vi "Set Current UUT.vi"(8 "error in (no error)":errorcluster, 10 "Current UUT":u32, 11 "LED Board Visual Test in":refnum<class "LED Board Test.lvclass">) -> (0 "error out":errorcluster, 3 "LED Board Visual Test out":refnum<class "LED Board Test.lvclass">)   [LabVIEW 2015, in "LED Board Test.lvclass"]
uses:
  LED Board Test.lvclass
  LED Board Test.lvclass/LED Board Test.ctl
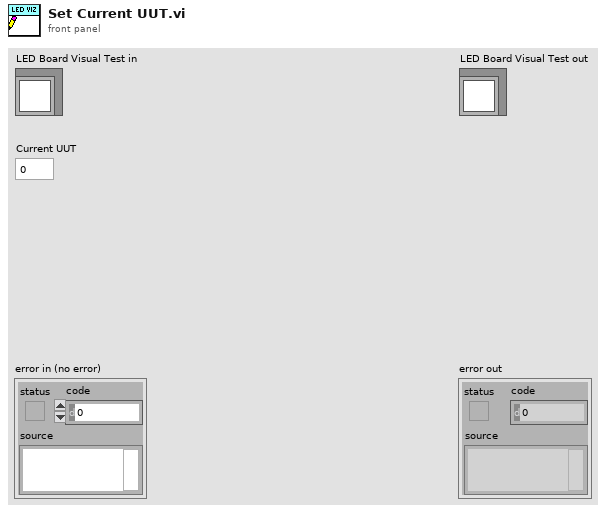
[diagram p1: front panel]
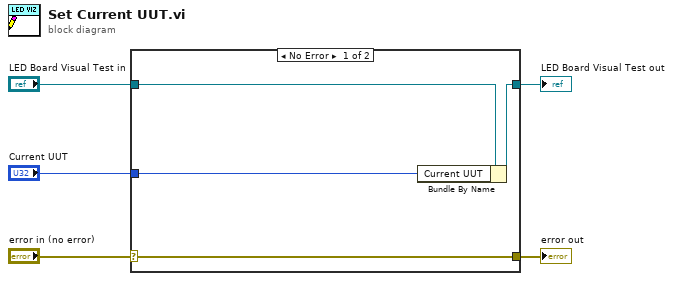
[diagram p0: block diagram]
diagram:
  n1 = case shown="No Error" "error in (no error)" {
    selector: "error in (no error)" -> [w9 w10]
    tunnel: [w9 w10] -> w4
    tunnel: [w7 w11] -> w2
    tunnel: "LED Board Visual Test in" -> [w8 w11]
    tunnel: "Current UUT" -> [w6 _]
    frame No Error {
      n2 = Bundle By Name(cluster=w8, "Current UUT"=w6) -> (w7:refnum<class "LED Board Test.lvclass">)
    }
    frame Error {
    }
  }
  "error out" <- w4
  "LED Board Visual Test out" <- w2
